vi "Read I32.vi"(8 "Error In":errorcluster, 11 "Reader In":refnum<class "Reader.lvclass">) -> (0 "Error Out":errorcluster, 2 "Value":i32, 3 "Reader Out":refnum<class "Reader.lvclass">)   [LabVIEW 2018, in "Toolkit.lvlib" / "Reader.lvclass"]
doc: "Reads and decodes a signed 32-bit integer from the MessagePack data."
uses:
  Reader.lvclass
  Reader.lvclass/Reader.ctl
  Status/Read Status.vi
  Status/Read Status Message.vi
  Status/Read Is Error.vi
  Utility/Status Code.vi
  <vilib>/Utility/error.llb/Error Cluster From Error Code.vi
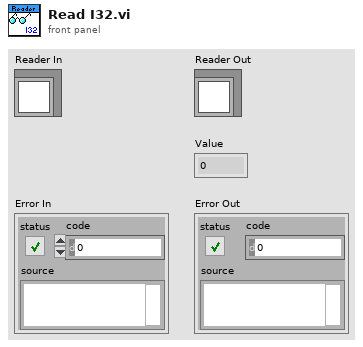
[diagram p1: front panel]
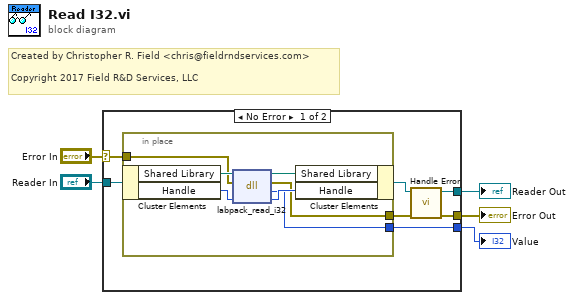
[diagram p0: block diagram]
diagram:
  # "Created by Christopher R. Field <chris@fieldrndservices.com>\n\nCopyright 2017 Field R&D Services, LLC"
  n1 = case shown="No Error" "Error In" {
    selector: "Error In" -> [w11 w20]
    tunnel: "Reader In" -> [w12 w21]
    tunnel: [w6 w20] -> w3
    tunnel: [w8 w21] -> w2
    tunnel: [w9 _] -> w1
    frame No Error {
      n2 = in-place {
        in-place-border: w11 -> [w15]
        in-place-border: [w14] -> w7
        in-place-border: [w13] -> w9
        n3 = in-place-cluster #1(w12) -> ("Shared Library"=w19:path, "Handle"=w17:u64)
        n4 = dll-call lib="D:/Users/cfield/Code/MessagePack/LabPack/LabVIEW/trunk/src/LabPack/Private/labpack-x64.dll" fn="labpack_read_i32"(path in=w19, error in=w15, "reader"=w17) -> (path out=w18:path, error out=w14:errorcluster, "return type"=w13:i32, "reader"=w16:u64)  [unwired: 1 in]
        n5 = in-place-cluster #1("Shared Library"=w18, "Handle"=w16) -> (w10:refnum<class "Reader.lvclass">)
      }
      n6 = call "Handle Error.vi"("Error In"=w7, "Reader In"=w10) -> ("Error Out"=w6:errorcluster, "Reader Out"=w8:refnum<class "Reader.lvclass">)  [unwired: 8 in]
    }
    frame Error {
    }
  }
  "Error Out" <- w3
  "Reader Out" <- w2
  "Value" <- w1
